vi "Generate Config File.vi"() -> ()   [LabVIEW 2013, in "About Screen Library.lvlib"]
uses:
  About Screen Library.lvlib
  Controls/Configuration Data.ctl
panel:
  in  "Cancel":bool
  in  "Window Title":string
  in  "Load Existing":bool
  in  "Background Color":u32(colorbox)
  out "error out":errorcluster
  in  "error in (no error)":errorcluster
  in  "Create Configuration File":bool
  in  "Load Existing Text":bool
  in  "Load Logo":bool
  in  "Load Banner":bool
  in  "Hyperlink":string
  in  "Include Hyperlink?":bool
  in  "About Text":string
  out "Logo (80 x 80)":picture
  out "Banner (720 x 80)":picture
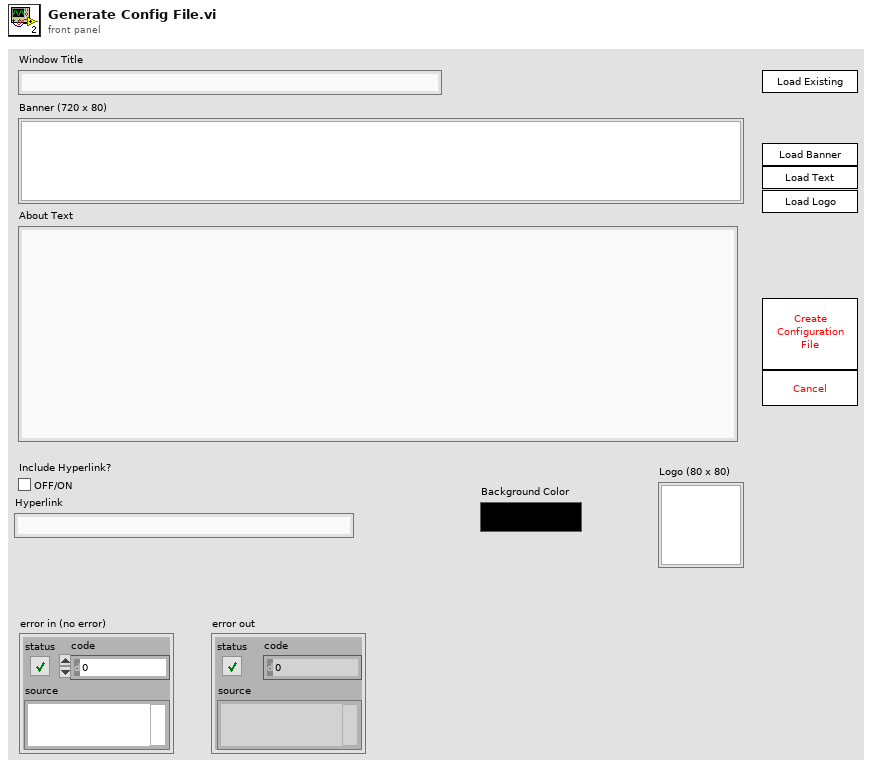
[diagram p1: front panel]
types:
  T1 = typedef "About Screen Library.lvlib/Configuration Data.ctl" = cluster{"Window Title":string, "About Text":string, "Include Hyperlink?":bool, "Hyperlink Path":string, "Logo (80 x 80)":picture, "Banner (720 x 80)":picture, "Background Color":u32}
  T2 = typedef "imagedata.ctl" = cluster{"image type":i32, "image depth":i32, "image":u8[], "mask":u8[], "colors":u32[], "Rectangle":cluster{"left":i16, "top":i16, "right":i16, "bottom":i16}}
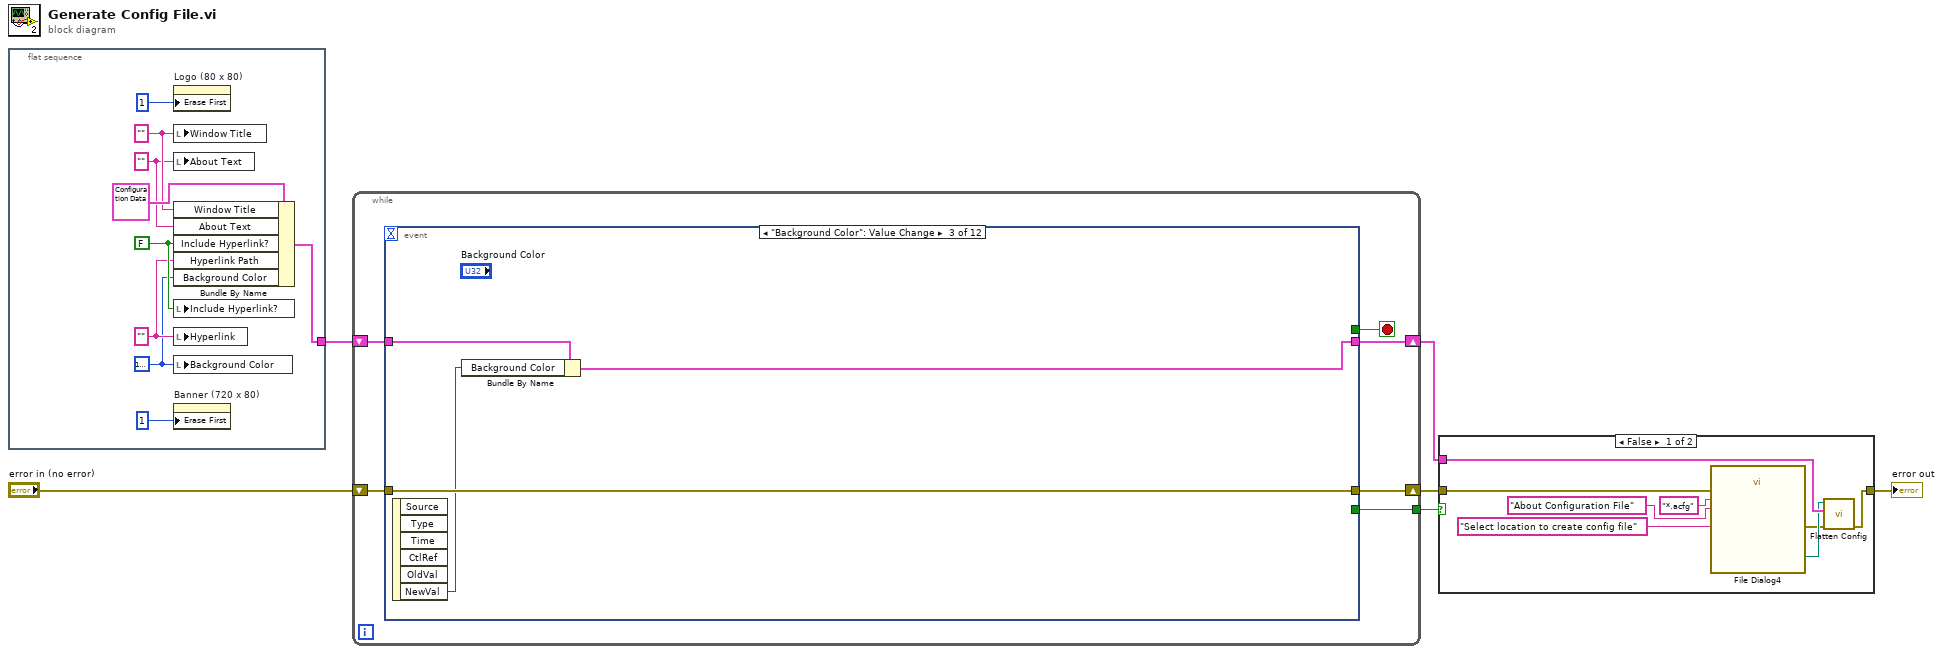
[diagram p0: block diagram]
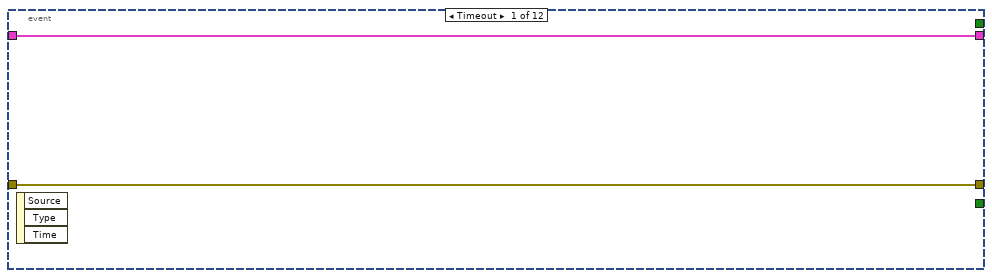
[diagram p3: hidden frame]
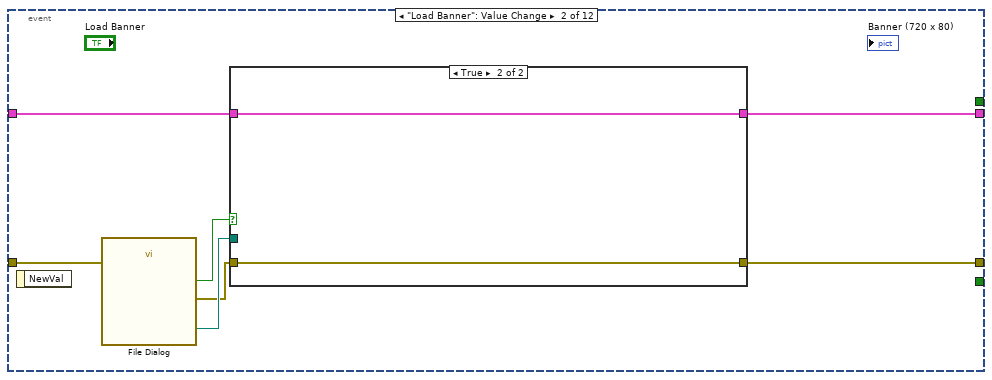
[diagram p4: hidden frame]
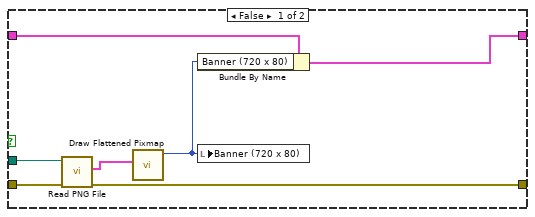
[diagram p5: hidden frame]
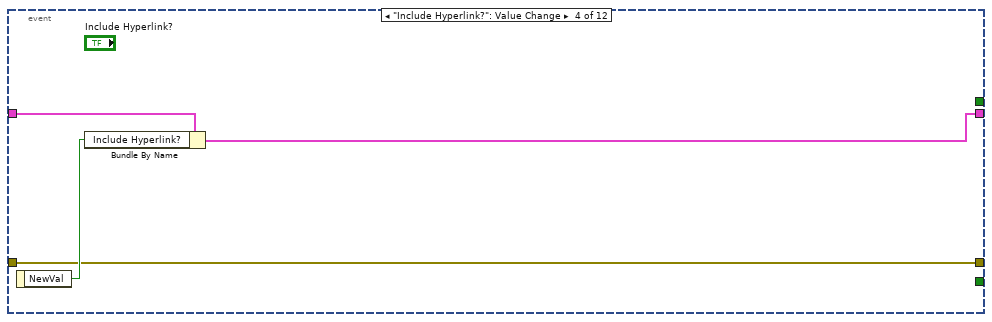
[diagram p6: hidden frame]
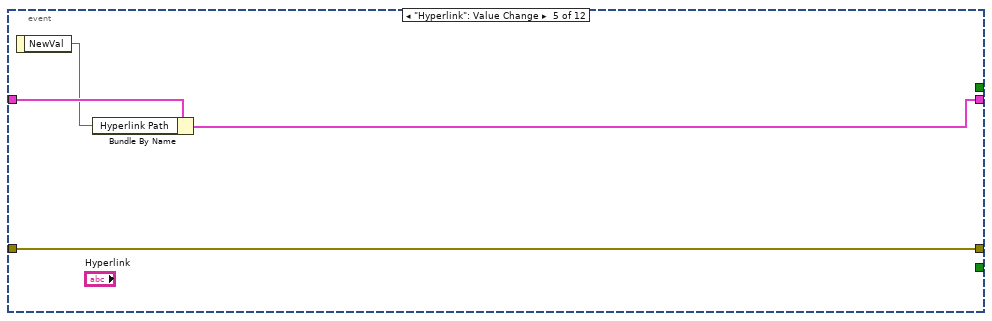
[diagram p7: hidden frame]
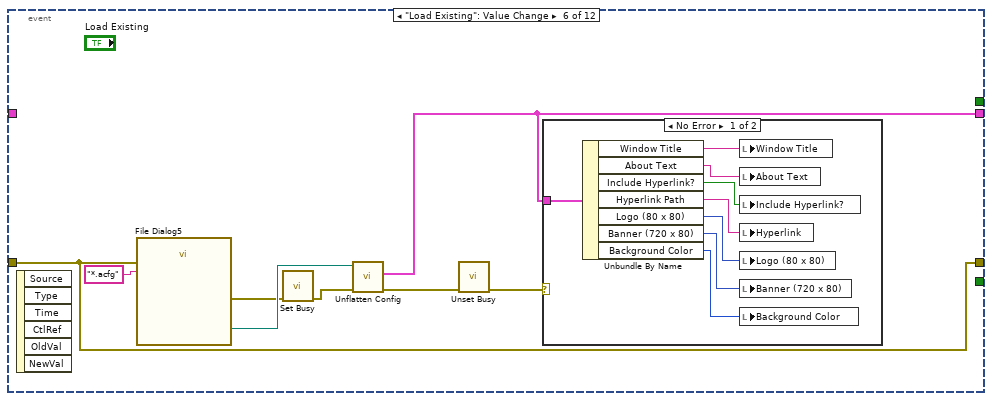
[diagram p8: hidden frame]
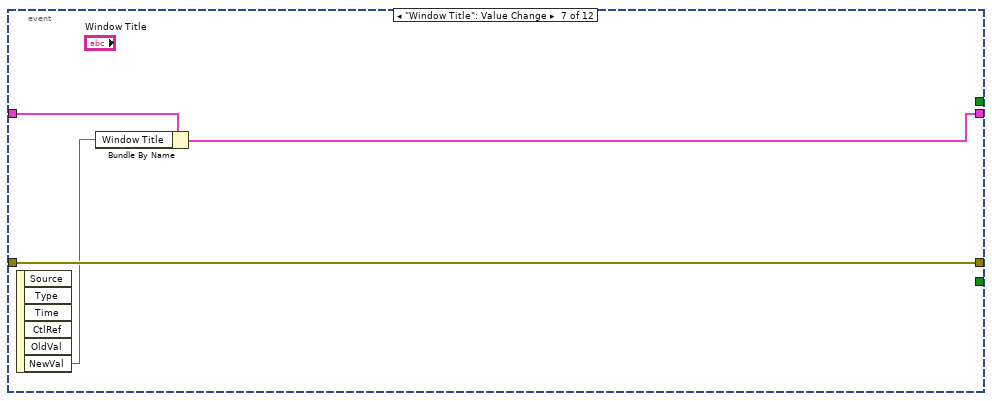
[diagram p10: hidden frame]
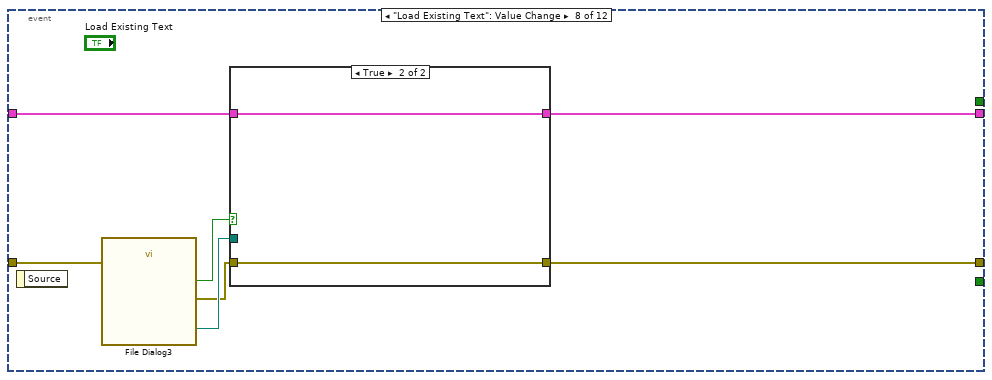
[diagram p11: hidden frame]
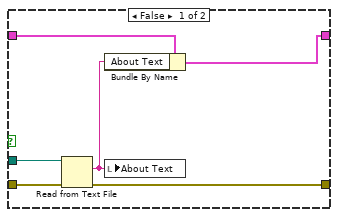
[diagram p12: hidden frame]
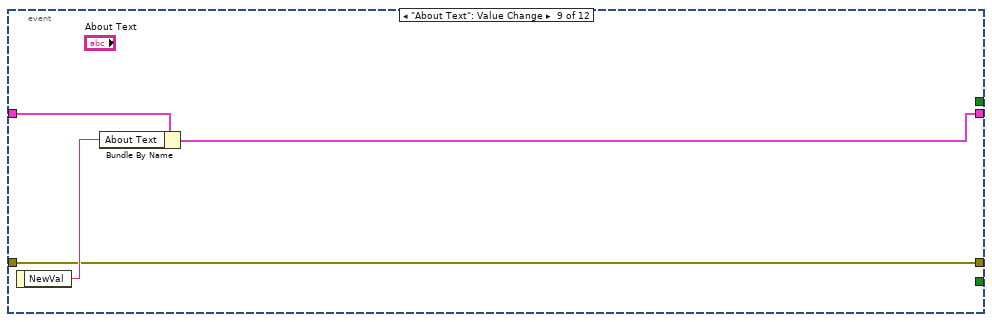
[diagram p13: hidden frame]
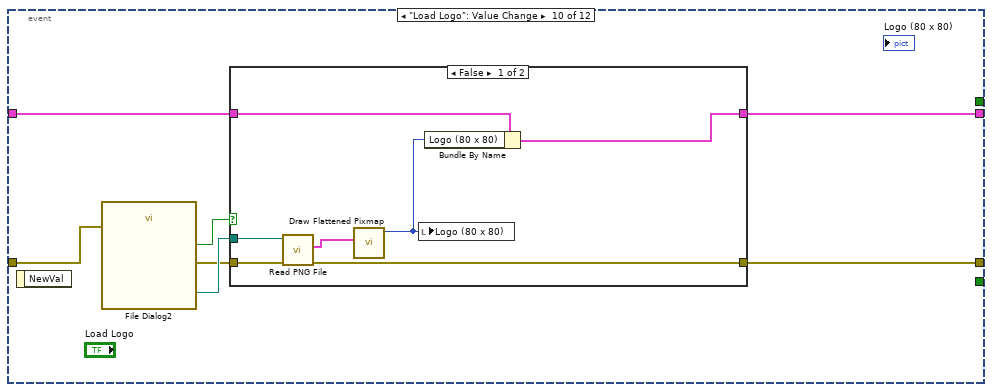
[diagram p14: hidden frame]
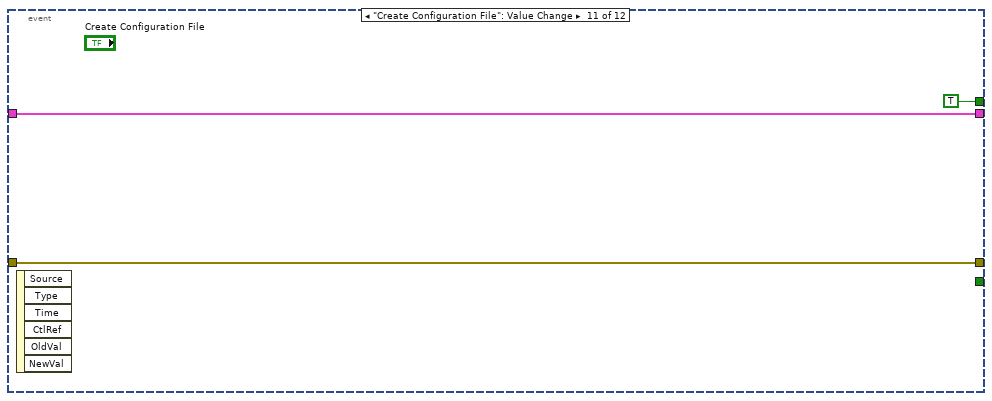
[diagram p16: hidden frame]
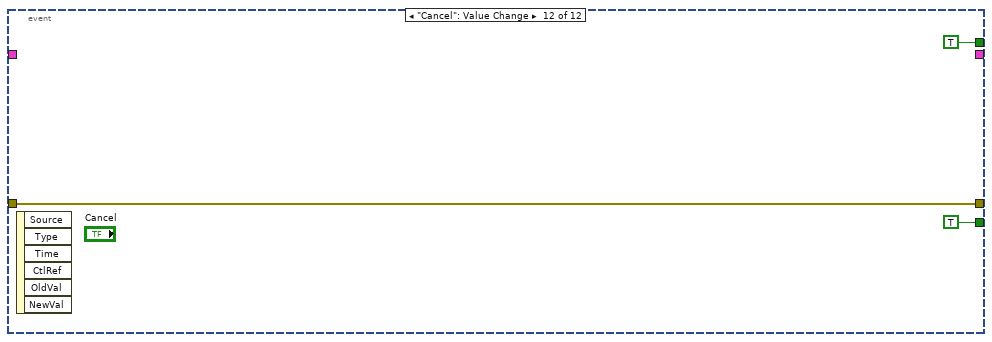
[diagram p17: hidden frame]
diagram:
  n1 = flat-sequence {
    tunnel: [w7] -> w6
    frame #0 {
      w12 = "" ("Window Title")
      w8 = u32 16777238 ("Background Color")
      w10 = FALSE ("Include Hyperlink?")
      w11 = "" ("About Text")
      w9 = "" ("Hyperlink")
      n2 = property on="Logo (80 x 80)" class="Pict"("Erase First"=u8 1) -> ()  [unwired: 2 in, 2 out]
      n3 = local write "Window Title"(w12) -> ()
      n4 = local write "About Text"(w11) -> ()
      n5 = Bundle By Name(cluster=T1 {"Window Title"="", "About Text"="", "Include Hyperlink?"=FALSE, "Hyperlink Path"="", "Logo (80 x 80)"=bytes[0], "Banner (720 x 80)"=bytes[0], "Background Color"=0} ("Configuration Data"), "Window Title"=w12, "About Text"=w11, "Include Hyperlink?"=w10, "Hyperlink Path"=w9, "Background Color"=w8) -> (w7:T1)
      n6 = local write "Include Hyperlink?"(w10) -> ()
      n7 = local write "Hyperlink"(w9) -> ()
      n8 = local write "Background Color"(w8) -> ()
      n9 = property on="Banner (720 x 80)" class="Pict"("Erase First"=u8 1) -> ()  [unwired: 2 in, 2 out]
    }
  }
  n10 = while {
    shift-right: [w19] -> w5
    shift-left: w6 -> [w20]
    shift-right: [w17] -> w3
    shift-left: "error in (no error)" -> [w18]
    tunnel: [w16] -> w1
    stop <- w21 stop-if-true
    n11 = event shown="[2] \"Background Color\": Value Change" {
      selector: _ -> [_ _ _ _ _ _ _ _ _ _ _ _]
      dyn-events: _ -> [_ _ _ _ _ _ _ _ _ _ _ _]
      timeout: _ -> [_ _ _ _ _ _ _ _ _ _ _ _]
      tunnel: [_ _ _ _ _ _ _ _ _ _ TRUE TRUE] -> w21
      tunnel: w20 -> [w23 w30 w42 w47 w51 _ w70 w77 w90 w97 w108 _]
      tunnel: [w23 w28 w40 w46 w49 w57 w68 w76 w89 w95 w108 _] -> w19
      tunnel: w18 -> [w22 w26 w43 w44 w48 w56 w71 w75 w87 w94 w107 w112]
      tunnel: [w22 w25 w43 w44 w48 w56 w71 w73 w87 w92 w107 w112] -> w17
      tunnel: [_ _ _ _ _ _ _ _ _ _ _ TRUE ("Cancel")] -> w16
      event Timeout {
        n12 = event-data() -> ()  [unwired: 1 in, 3 out]
      }
      event "Load Banner": Value Change {
        n13 = event-data() -> ()  [unwired: 1 in, 1 out]
        n14 = call "File Dialog"("error in"=w26) -> ("selected path"=w29:path, "cancelled"=w24:bool, "error out"=w27:errorcluster)  [unwired: 11 in, 1 out]
        n15 = case shown="True" w24 {
          tunnel: w30 -> [w37 w39]
          tunnel: w29 -> [w36 _]
          tunnel: [w35 w39] -> w28
          tunnel: w27 -> [w33 w38]
          tunnel: [w32 w38] -> w25
          frame False {
            n16 = call <vilib>:"Read PNG File.vi"("error in (no error)"=w33, "path to PNG file"=w36) -> ("error out"=w32:errorcluster, "image data"=w34:T2)  [unwired: 7 in, 1 out]
            n17 = call <vilib>:"Draw Flattened Pixmap.vi"("image data"=w34) -> ("new picture"=w31:picture)  [unwired: 8 in]
            n18 = Bundle By Name(cluster=w37, "Banner (720 x 80)"=w31) -> (w35:T1)
            n19 = local write "Banner (720 x 80)"(w31) -> ()
          }
          frame True {
          }
        }
      }
      event "Background Color": Value Change {
        n20 = event-data() -> ("NewVal"=w41:u32)  [unwired: 1 in, 5 out]
        n21 = Bundle By Name(cluster=w42, "Background Color"=w41) -> (w40:T1)
      }
      event "Include Hyperlink?": Value Change {
        n22 = event-data() -> ("NewVal"=w45:bool)  [unwired: 1 in]
        n23 = Bundle By Name(cluster=w47, "Include Hyperlink?"=w45) -> (w46:T1)
      }
      event "Hyperlink": Value Change {
        n24 = event-data() -> ("NewVal"=w50:string)  [unwired: 1 in]
        n25 = Bundle By Name(cluster=w51, "Hyperlink Path"=w50) -> (w49:T1)
      }
      event "Load Existing": Value Change {
        n26 = event-data() -> ()  [unwired: 1 in, 6 out]
        n27 = call "File Dialog5"("error in"=w56, "pattern (all files)"="*.acfg") -> ("selected path"=w58:path, "error out"=w55:errorcluster)  [unwired: 10 in, 2 out]
        n28 = call <vilib>:"Set Busy.vi"("error in (no error)"=w55) -> ("error out"=w54:errorcluster)  [unwired: 9 in, 1 out]
        n29 = call "Unflatten Config.vi"("error in (no error)"=w54, "About Configuration File"=w58) -> ("error out"=w53:errorcluster, "About Configuration"=w57:T1)  [unwired: 8 in]
        n30 = call <vilib>:"Unset Busy.vi"("error in (no error)"=w53) -> ("error out"=w52:errorcluster)  [unwired: 10 in]
        n31 = case shown="No Error" w52 {
          tunnel: w57 -> [w67 _]
          frame No Error {
            n32 = Unbundle By Name(w67) -> ("Window Title"=w60:string, "About Text"=w66:string, "Include Hyperlink?"=w65:bool, "Hyperlink Path"=w64:string, "Logo (80 x 80)"=w63:picture, "Banner (720 x 80)"=w62:picture, "Background Color"=w61:u32)
            n33 = local write "Window Title"(w60) -> ()
            n34 = local write "About Text"(w66) -> ()
            n35 = local write "Include Hyperlink?"(w65) -> ()
            n36 = local write "Hyperlink"(w64) -> ()
            n37 = local write "Logo (80 x 80)"(w63) -> ()
            n38 = local write "Banner (720 x 80)"(w62) -> ()
            n39 = local write "Background Color"(w61) -> ()
          }
          frame Error {
          }
        }
      }
      event "Window Title": Value Change {
        n40 = event-data() -> ("NewVal"=w69:string)  [unwired: 1 in, 5 out]
        n41 = Bundle By Name(cluster=w70, "Window Title"=w69) -> (w68:T1)
      }
      event "Load Existing Text": Value Change {
        n42 = event-data() -> ()  [unwired: 1 in, 1 out]
        n43 = call "File Dialog3"("error in"=w75) -> ("selected path"=w78:path, "cancelled"=w72:bool, "error out"=w74:errorcluster)  [unwired: 11 in, 1 out]
        n44 = case shown="True" w72 {
          tunnel: w78 -> [w84 _]
          tunnel: w77 -> [w83 w86]
          tunnel: [w81 w86] -> w76
          tunnel: w74 -> [w80 w85]
          tunnel: [w79 w85] -> w73
          frame False {
            n45 = Read from Text File(file (use dialog)=w84, error in=w80) -> (text=w82:string, error out=w79:errorcluster)  [unwired: 2 in, 2 out]
            n46 = Bundle By Name(cluster=w83, "About Text"=w82) -> (w81:T1)
            n47 = local write "About Text"(w82) -> ()
          }
          frame True {
          }
        }
      }
      event "About Text": Value Change {
        n48 = event-data() -> ("NewVal"=w88:string)  [unwired: 1 in]
        n49 = Bundle By Name(cluster=w90, "About Text"=w88) -> (w89:T1)
      }
      event "Load Logo": Value Change {
        n50 = event-data() -> ()  [unwired: 1 in, 1 out]
        n51 = call "File Dialog2"("error in"=w94) -> ("selected path"=w96:path, "cancelled"=w91:bool, "error out"=w93:errorcluster)  [unwired: 11 in, 1 out]
        n52 = case shown="False" w91 {
          tunnel: w97 -> [w104 w106]
          tunnel: w96 -> [w103 _]
          tunnel: [w102 w106] -> w95
          tunnel: w93 -> [w100 w105]
          tunnel: [w99 w105] -> w92
          frame False {
            n53 = call <vilib>:"Read PNG File.vi"("error in (no error)"=w100, "path to PNG file"=w103) -> ("error out"=w99:errorcluster, "image data"=w101:T2)  [unwired: 7 in, 1 out]
            n54 = call <vilib>:"Draw Flattened Pixmap.vi"("image data"=w101) -> ("new picture"=w98:picture)  [unwired: 8 in]
            n55 = local write "Logo (80 x 80)"(w98) -> ()
            n56 = Bundle By Name(cluster=w104, "Logo (80 x 80)"=w98) -> (w102:T1)
          }
          frame True {
          }
        }
      }
      event "Create Configuration File": Value Change {
        n57 = event-data() -> ()  [unwired: 1 in, 6 out]
      }
      event "Cancel": Value Change {
        n58 = event-data() -> ()  [unwired: 1 in, 6 out]
      }
    }
  }
  n59 = case shown="False" w1 {
    tunnel: w5 -> [w119 _]
    tunnel: w3 -> [w117 w121]
    tunnel: [w115 w121] -> w2
    frame False {
      n60 = call "File Dialog4"("prompt"="Select location to create config file", "error in"=w117, "pattern (all files)"="*.acfg" ("pattern label"), "pattern label"="About Configuration File") -> ("selected path"=w118:path, "error out"=w116:errorcluster)  [unwired: 8 in, 2 out]
      n61 = call "Flatten Config.vi"("error in (no error)"=w116, "Configuration Data"=w119, "selected path"=w118) -> ("error out"=w115:errorcluster)  [unwired: 8 in]
    }
    frame True {
    }
  }
  "error out" <- w2
